vi "123.vi"(8 "error IO 2":errorcluster, 9 "T min":dbl format="%#_13g", 10 "T Max":dbl format="%#_13g", 11 "T":dbl format="%#_13g") -> (1 "error IO":errorcluster, 2 "String":string, 3 "Warning":bool)   [LabVIEW 2015]
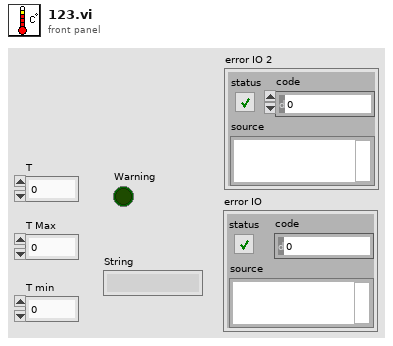
[diagram p1: front panel]
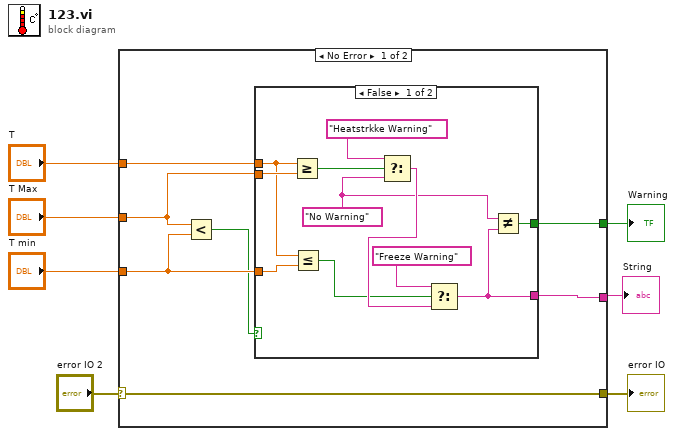
[diagram p0: block diagram]
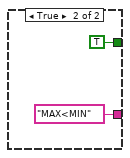
[diagram p2: hidden frame]
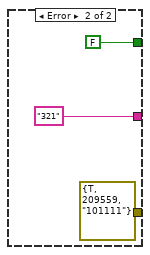
[diagram p3: hidden frame]
diagram:
  n1 = case shown="No Error" "error IO 2" {
    selector: "error IO 2" -> [w10 _]
    tunnel: "T" -> [w14 _]
    tunnel: "T Max" -> [w8 _]
    tunnel: "T min" -> [w13 _]
    tunnel: [w12 "321" ("String 2")] -> w3
    tunnel: [w11 FALSE] -> w4
    tunnel: [w10 errorcluster {"status"=TRUE, "code"=209559, "source"="101111"} ("error IO")] -> w2
    frame No Error {
      n2 = Less?(x=w8, y=w13) -> (x < y?=w9:bool)
      n3 = case shown="False" w9 {
        tunnel: w14 -> [w23 _]
        tunnel: w8 -> [w25 _]
        tunnel: w13 -> [w24 _]
        tunnel: [w16 "MAX<MIN"] -> w12
        tunnel: [w15 TRUE] -> w11
        frame False {
          w17 = "No Warning"
          n4 = Greater Or Equal?(x=w23, y=w25) -> (x >= y?=w22:bool)
          n5 = Less Or Equal?(x=w23, y=w24) -> (x <= y?=w18:bool)
          n6 = Select(t="Heatstrkke Warning", s=w22, f=w17) -> (s? t:f=w19:string)
          n7 = Select(t="Freeze Warning", s=w18, f=w19) -> (s? t:f=w16:string)
          n8 = Not Equal?(x=w17, y=w16) -> (x != y?=w15:bool)
        }
        frame True {
        }
      }
    }
    frame Error {
    }
  }
  "Warning" <- w4
  "String" <- w3
  "error IO" <- w2
